vi "in_spline y1 to coefficients.vi"(9 "Y1":dbl[](array[numeric]), 10 "X":dbl[](array[numeric]), 11 "Y":dbl[](array[numeric])) -> (3 "coefficients":dbl[][](array[numeric]))   [LabVIEW 2014, in "NI_Gmath.lvlib"]
uses:
  NI_Gmath.lvlib
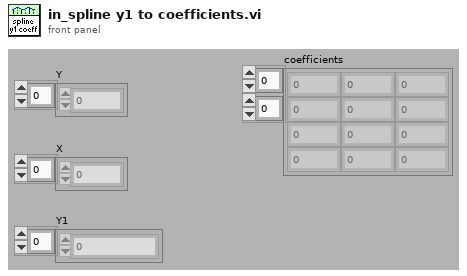
[diagram p1: front panel]
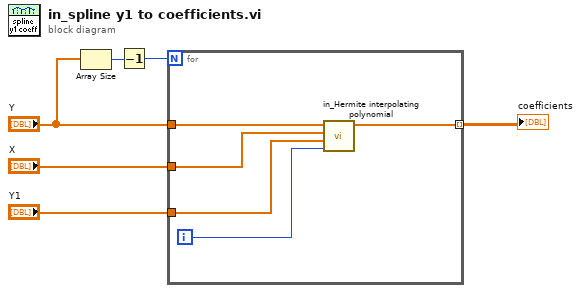
[diagram p0: block diagram]
diagram:
  n1 = Array Size(array="Y") -> (size(s)=w5:i32)
  n2 = Decrement(x=w5) -> (x-1=w4:i32)
  n3 = for {
    N: w4 -> [_]
    tunnel: "Y" -> [w11]
    tunnel: "X" -> [w10]
    tunnel: "Y1" -> [w9]
    tunnel: [w7] -> w2 mode=indexing
    i -> [w8]
    n4 = call "in_Hermite interpolating polynomial.vi"("index i"=w8, "Y deriv[0..N]"=w9, "X[0..N]"=w10, "Y[0..N]"=w11) -> ("Hermite polynomial"=w7:dbl[])  [unwired: 7 in]
  }
  "coefficients" <- w2
